vi "test Add Alias To Empty List.vi"(8 "error in (no error)":errorcluster, 11 "TestCase in":refnum<class "Routing and Faulting Aliases Unit Tests.lvclass">) -> (0 "error out":errorcluster, 3 "TestCase out":refnum<class "Routing and Faulting Aliases Unit Tests.lvclass">)   [LabVIEW 2017, in "Routing and Faulting Aliases Unit Tests.lvclass"]
uses:
  Routing and Faulting Aliases Unit Tests.lvclass
  System Explorer/Alias.ctl
  System Explorer/Endpoint.ctl
  Shared/Alias Mapping.ctl
  Routing and Faulting Aliases Unit Tests.lvclass/Routing and Faulting Aliases Unit Tests.ctl
  <vilib>/addons/_JKI Toolkits/VI Tester/TestCase.llb/TestCase.lvclass
  System Explorer/Routing and Faulting System Explorer.lvlib
  Scripting/Routing and Faulting Scripting.lvlib
  Shared/Routing and Faulting Shared.lvlib
  C:/Program Files (x86)/National Instruments/LabVIEW 2017/vi.lib/addons/_JKI Toolkits/VI Tester/TestCase.llb/TestCase.lvclass
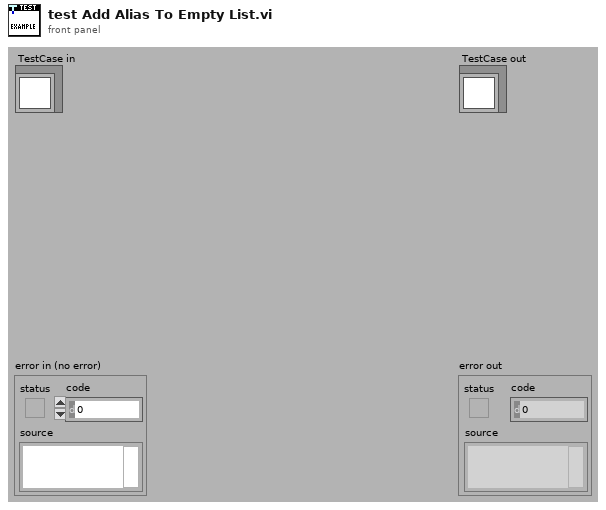
[diagram p1: front panel]
types:
  T1 = typedef "Routing and Faulting Shared.lvlib/Alias Mapping.ctl" = cluster{"Endpoint":string, "Alias":string}
  T2 = typedef "Routing and Faulting System Explorer.lvlib/Alias.ctl" = cluster{"Endpoint":T3, "Alias":string, "Remove":bool}
  T3 = typedef "Routing and Faulting System Explorer.lvlib/Endpoint.ctl" = string
  T4 = typedef "Custom Device API.lvlib/Custom Device Item Ref.ctl" = u64
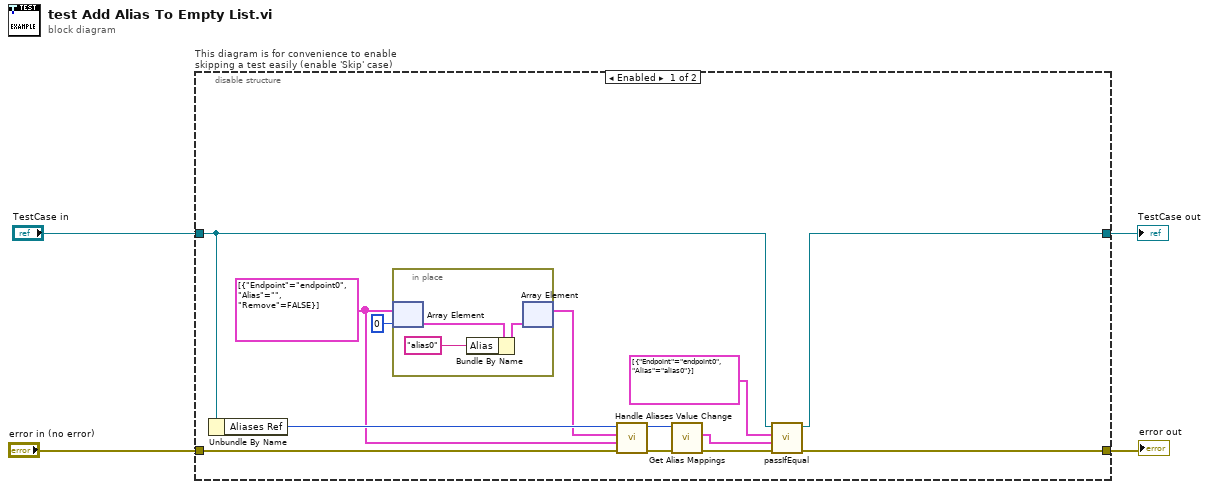
[diagram p0: block diagram]
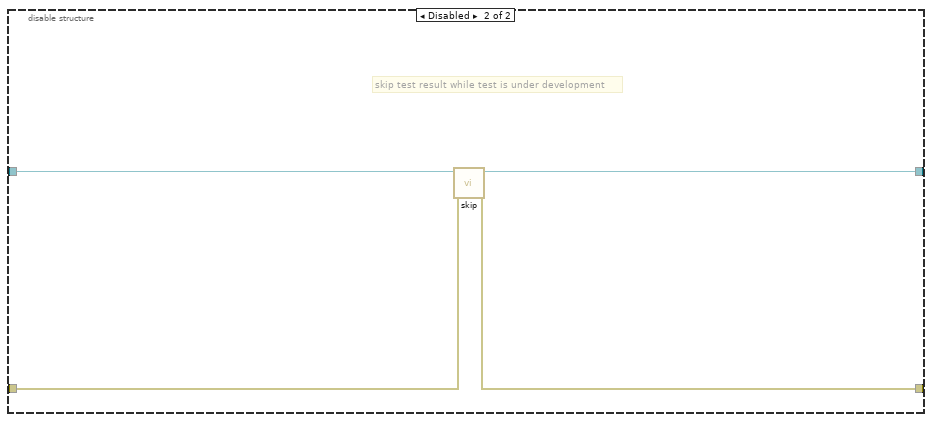
[diagram p2: hidden frame]
diagram:
  n1 = disable-structure "This diagram is for convenience to enable skipping a test easily (enable 'Skip' case)" shown="Enabled" {
    disable-tunnel: "TestCase in" -> [w9 w24]
    disable-tunnel: [w8 w22] -> w1
    disable-tunnel: [w12 w23] -> w3
    disable-tunnel: "error in (no error)" -> [w17 w21]
    frame Enabled {
      w7 = T2[] [{"Endpoint"="endpoint0", "Alias"="", "Remove"=FALSE}] ("NewVal")
      n2 = Unbundle By Name(w9) -> ("Aliases Ref"=w16:T4)
      n3 = in-place {
        n4 = in-place-array #1(w7, 0) -> (w20:T2)
        n5 = Bundle By Name(cluster=w20, "Alias"="alias0") -> (w19:T2)
        n6 = in-place-array #1(w19) -> (w6:T2[])  [unwired: 1 out]
      }
      n7 = call "Handle Aliases Value Change.vi"("error in (no error)"=w17, "OldVal"=w7, "NewVal"=w6, "Aliases Ref in"=w16) -> ("error out"=w15:errorcluster, "Aliases Ref out"=w14:T4)  [unwired: 6 in]
      n8 = call "Get Alias Mappings.vi"("error in (no error)"=w15, "Endpoint Aliases Ref in"=w14) -> ("error out"=w13:errorcluster, "Alias Mappings"=w11:T1[])  [unwired: 7 in, 1 out]
      n9 = call-dynamic "passIfEqual.vi"("error in (no error)"=w13, "y"=w11, "x"=T1[] [{"Endpoint"="endpoint0", "Alias"="alias0"}] ("Alias Mappings"), "TestCase in"=w9) -> ("error out"=w12:errorcluster, "TestCase out"=w8:refnum<class "Routing and Faulting Aliases Unit Tests.lvclass">)  [unwired: 6 in]
    }
    frame Disabled {
      # "skip test result while test is under development"
      n10 = call <vilib>:"skip.vi"("error in (no error)"=w21, "TestCase in"=w24) -> ("error out"=w23:errorcluster, "TestCase out"=w22:refnum<class "Routing and Faulting Aliases Unit Tests.lvclass">)  [unwired: 8 in]
    }
  }
  "error out" <- w3
  "TestCase out" <- w1
